vi "Mass-Flow Controller.vi"() -> ()   [LabVIEW 2018]
uses:
  <vilib>/addons/control/pid/pid.llb/PID Gain Schedule (DBL).vi
  <vilib>/addons/control/pid/pid.llb/PID Advanced (DBL).vi
  <vilib>/addons/control/pid/NI_PID_pid.lvlib
panel:
  out "Scaled MV":dbl(slide) scale=0.0..2000.0
  in  "stop":bool
  in  "PID gain schedule":T1(array[cluster])=[{"PID gains"={"proportional gain (Kc)"=1.0, "integral time (Ti, min)"=0.01, "derivative time (Td, min)"=0.0}, "max value"=100.0}] {"max value" format="%.2f"; "PID gains"."derivative time (Td, min)" format="%.6f"; "PID gains"."integral time (Ti, min)" format="%.6f"; "PID gains"."proportional gain (Kc)" format="%.6f"}
  in  "Sampling Time dt (s)":dbl=0.05 min=0.001 step=0.01 format="%#.3p"
  in  "Pressure Readout (in Torr)":dbl
  in  "Target Pressure(in Torr)":dbl
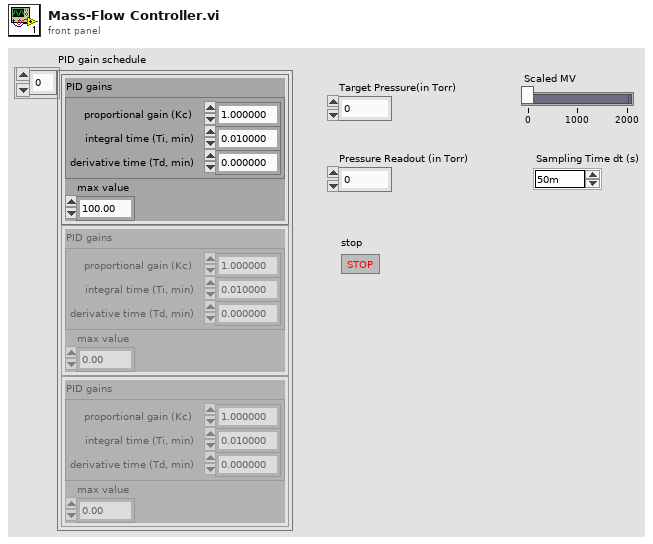
[diagram p1: front panel]
types:
  T1 = cluster{"PID gains":cluster{"proportional gain (Kc)":dbl, "integral time (Ti, min)":dbl, "derivative time (Td, min)":dbl}, "max value":dbl}[]
  T2 = cluster{"proportional gain (Kc)":dbl, "integral time (Ti, min)":dbl, "derivative time (Td, min)":dbl}
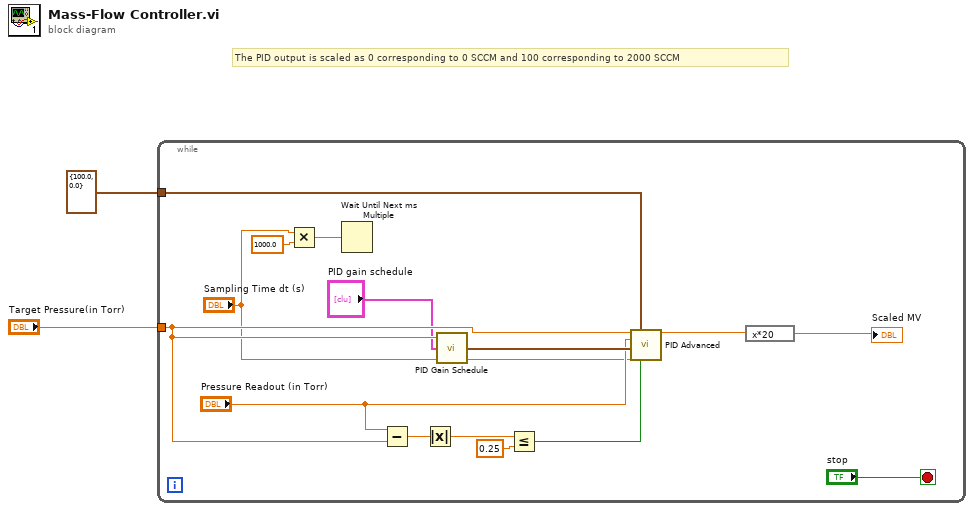
[diagram p0: block diagram]
diagram:
  # "The PID output is scaled as 0 corresponding to 0 SCCM and 100 corresponding to 2000 SCCM"
  n1 = while {
    tunnel: cluster{"output high":dbl, "output low":dbl} {"output high"=100.0, "output low"=0.0} ("output range") -> [w17]
    tunnel: "Target Pressure(in Torr)" -> [w11]
    stop <- "stop" stop-if-true
    n2 = Multiply(x="Sampling Time dt (s)", y=1000.0) -> (x*y=w9:dbl)
    n3 = Wait Until Next ms Multiple(millisecond multiple=w9) -> ()  [unwired: 1 out]
    n4 = Subtract(x="Pressure Readout (in Torr)", y=w11) -> (x-y=w15:dbl)
    n5 = Absolute Value(x=w15) -> (abs(x)=w14:dbl)
    n6 = call-poly <vilib>:"PID Gain Schedule.vi"("PID gain schedule"="PID gain schedule", "gain scheduling value"=w11) -> ("PID gains out"=w16:T2)  [unwired: 2 in, 1 out]
    n7 = Less Or Equal?(x=w14, y=0.25) -> (x <= y?=w10:bool)
    n8 = call-poly <vilib>:"PID Advanced.vi"("setpoint"=w11, "output range"=w17, "process variable"="Pressure Readout (in Torr)", "PID gains"=w16, "dt (s)"="Sampling Time dt (s)", "reinitialize? (F)"=w10) -> ("output"=w4:dbl)  [unwired: 8 in, 1 out]
    n9 = expression code="x*20"(w4) -> (→"Scaled MV":dbl)
  }
